vi "Menu_Toggle.vi"(8 "error in (no error)":errorcluster, 10 "item tag":string, 11 "menu":refnum<k9>) -> (0 "error out":errorcluster, 1 "state":bool, 3 "dup menu":refnum<k9>)   [LabVIEW 2011]
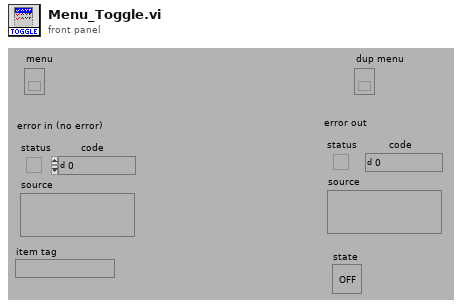
[diagram p1: front panel]
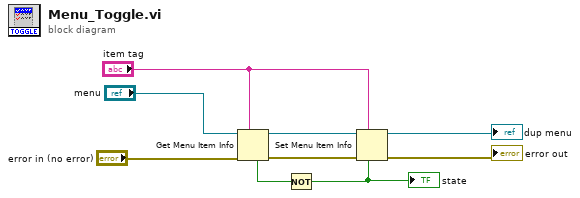
[diagram p0: block diagram]
diagram:
  n1 = Get Menu Item Info(7:"item tag", 8:"error in (no error)", 11:"menu") -> (0:w8:errorcluster, 3:w4:refnum<k9>, 4:w3:bool)  [unwired: 4 out]
  n2 = Not(x=w3) -> (.not. x?=w2:bool)
  "state" <- w2
  n3 = Set Menu Item Info(6:w2, 7:"item tag", 8:w8, 11:w4) -> (0:→"error out":errorcluster, 3:→"dup menu":refnum<k9>)  [unwired: 3 in]
